vi "FollowPath.vi"(1 "Parameter String":string, 2 "Reinit":bool) -> (0 "Increment":bool)   [LabVIEW 2018]
uses:
  sensors.vi
  refnums.vi
  <vilib>/Rock Robotics/WPI/Utilities/WPI_GetSetVariantRefNum.vi
  dsinstructions.vi
panel:
  out "Robot Position":cluster{dbl[], dbl[]}[](graph)
  in  "Plot":bool
  in  "N-Int":i32=50
  in  "N-Diff":i32=50
  in  "Kd":dbl=1e-06
  in  "Ki":dbl=5e-06
  in  "Kp":dbl=3e-05
  out "Orientation PID Tracking":cluster{"Goal Wheel Position":dbl, dbl}(graph)={"Goal Wheel Position"=0.0, -90.17571233858979}
  out "Orientation Contribution Tracking":cluster{dbl, dbl, dbl}(graph)
  in  "Manual Control":bool=TRUE
  in  "Look-Ahead Time (s)":dbl=0.25
  in  "Search Window (s)":dbl=2.0
  # "Orientation Control"
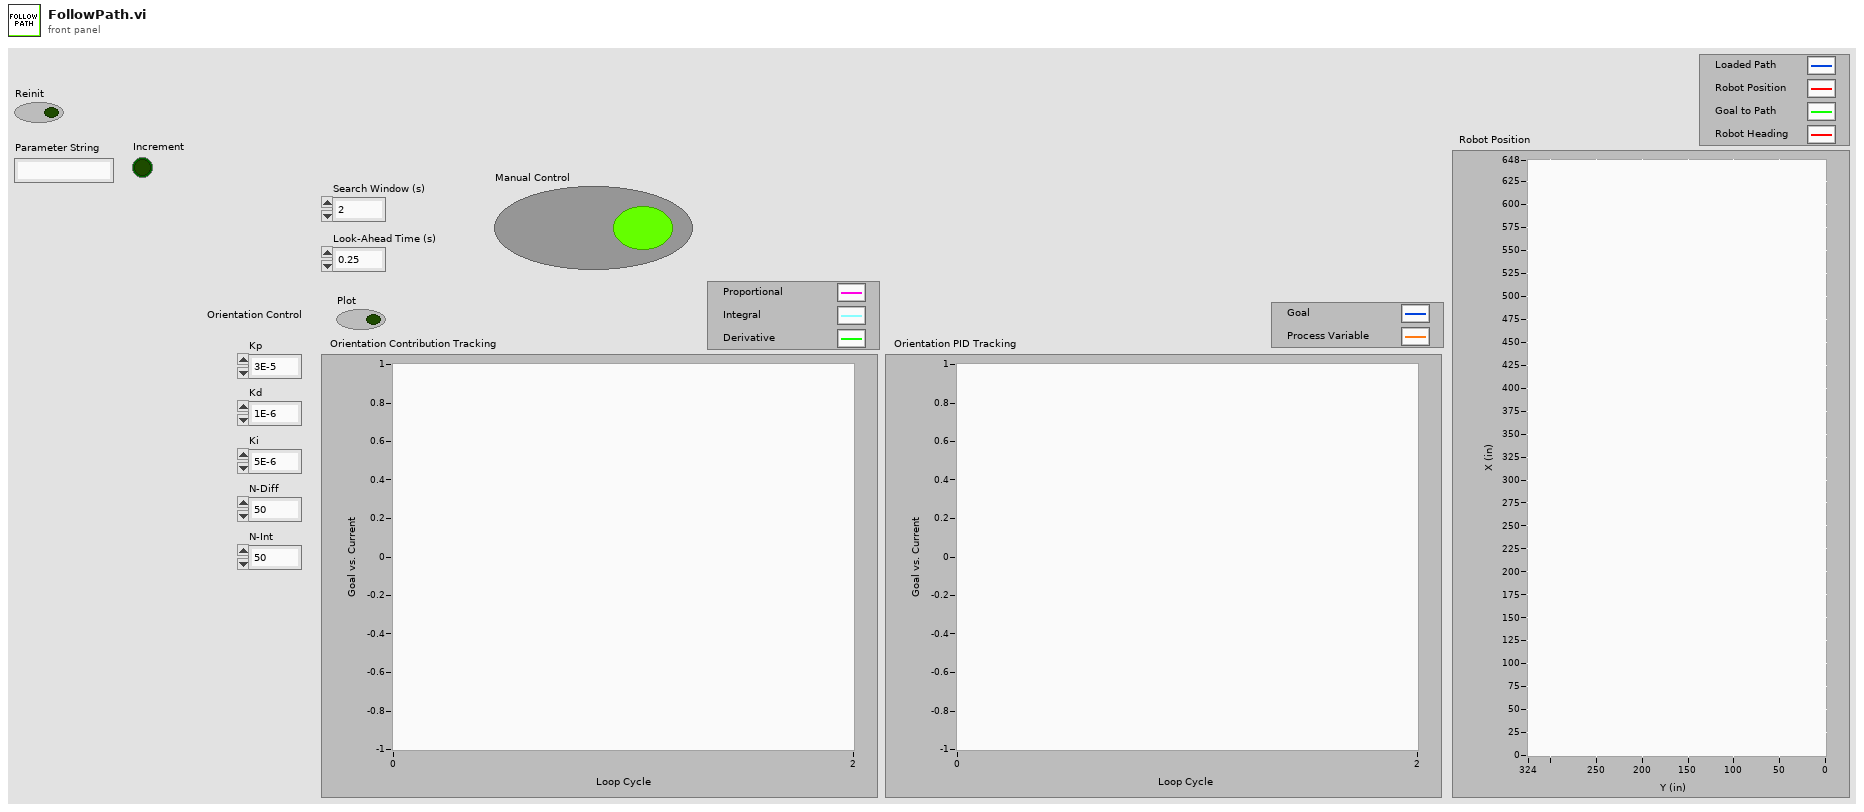
[diagram p1: front panel]
types:
  T1 = typedef "WPI_JoystickDevRef.ctl" = cluster{"Device":T2}
  T2 = typedef "WPI_JoystickDeviceEnum.ctl" = enum16{"USB 0", "USB 1", "USB 2", "USB 3", "USB 4", "USB 5"}
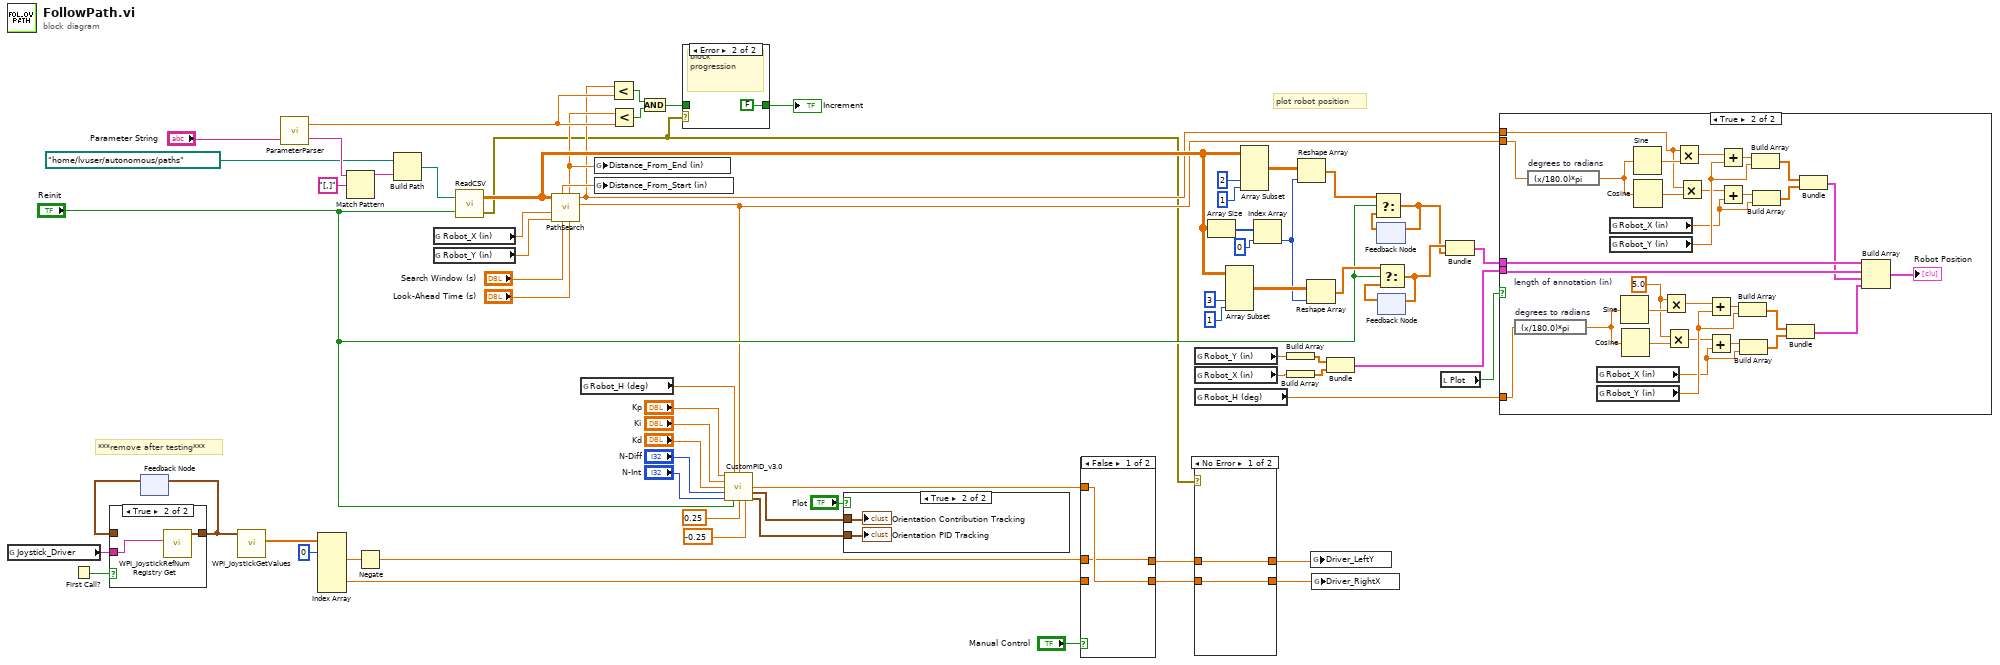
[diagram p0: block diagram]
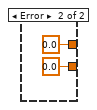
[diagram p3: hidden frame]
diagram:
  # "***remove after testing***"
  # "plot robot position"
  n1 = global read "refnums.vi" "Joystick_Driver"() -> (w57:string)
  n2 = First Call?() -> (First Call?: T/F=w60:bool)
  n3 = feedback #1() -> (w59:T1)  [unwired: 1 in]
  n4 = case shown="True" w60 {
    tunnel: [w72 w74] -> w58
    tunnel: w59 -> [w72 _]
    tunnel: w57 -> [_ w73]
    frame False {
    }
    frame True {
      n5 = call <vilib>:"WPI_JoystickRefNum Registry Get.vi"("refnum name"=w73) -> ("JoystickDevRef"=w74:T1)  [unwired: 9 in, 1 out]
    }
  }
  n6 = feedback-in #1(w58) -> ()
  n7 = call <vilib>:"WPI_JoystickGetValues.vi"("JoystickDevRef"=w58) -> ("Axes"=w56:dbl[])  [unwired: 6 in, 4 out]
  n8 = call "ParameterParser.vi"("Parameter String"="Parameter String") -> ("Remaining Parameter String"=w69:string, "Parameter"=w11:dbl)  [unwired: 1 in]
  n9 = Index Array(array=w56, index #1=0 ("index")) -> (element #2=w54:dbl, element #5=w52:dbl)  [unwired: 5 in, 4 out]
  n10 = Match Pattern(string=w69, regular expression="[,]") -> (before substring=w68:string)  [unwired: 1 in, 3 out]
  n11 = Negate(x=w54) -> (-x=w53:dbl)
  n12 = Build Path(base path=path "/home/lvuser/autonomous/paths" ("path"), name or relative path=w68) -> (appended path=w66:path)
  n13 = global read "sensors.vi" "Robot_X (in)"() -> (w64:dbl)
  n14 = global read "sensors.vi" "Robot_Y (in)"() -> (w63:dbl)
  n15 = call "ReadCSV.vi"("Reinit"="Reinit", "File Path (.csv)"=w66) -> ("File Open Eror"=w4:errorcluster, "Data (index by row)"=w26:dbl[][])
  n16 = call "PathSearch.vi"("Look-Ahead Time (s)"="Look-Ahead Time (s)", "Search Window (s)"="Search Window (s)", "Robot Y (in)"=w63, "Robot X (in)"=w64, "Path"=w26) -> ("Angle To Goal (deg)"=w12:dbl, "Distance to Goal (in)"=w9:dbl, "Distance from End (in)"=w10:dbl, "Distance from Start (in)"=w65:dbl)  [unwired: 1 in, 2 out]
  n17 = global read "sensors.vi" "Robot_H (deg)"() -> (w50:dbl)
  n18 = global write "sensors.vi" "Distance_From_End (in)"(w10) -> ()
  n19 = global write "sensors.vi" "Distance_From_Start (in)"(w65) -> ()
  n20 = Less?(x=w9, y=w11) -> (x < y?=w28:bool)
  n21 = Less?(x=w10, y=w11) -> (x < y?=w27:bool)
  n22 = And(x=w28, y=w27) -> (x .and. y?=w3:bool)
  n23 = case shown="Error" w4 {
    tunnel: [w75 FALSE] -> w2
    tunnel: w3 -> [w75 _]
    frame No Error {
    }
    frame Error {
      # "block progression"
    }
  }
  "Increment" <- w2
  n24 = call "CustomPID_v3.0.vi"("Kp"="Kp", "Process Variable"=w50, "Goal"=w12, "Ki"="Ki", "Kd"="Kd", "N-Diff"="N-Diff", "N-Int"="N-Int", "Reinit"="Reinit", "Max Ouput"=0.25, "Min Output"=-0.25) -> ("Command"=w49:dbl, "Contribution Tracking"=w48:cluster{dbl, dbl, dbl}, "PID Tracking"=w47:cluster{"Goal Wheel Position":dbl, dbl})  [unwired: 2 in, 1 out]
  n25 = case shown="True" "Plot" {
    tunnel: w48 -> [_ w78]
    tunnel: w47 -> [_ w77]
    frame False {
    }
    frame True {
      "Orientation Contribution Tracking" <- w78
      "Orientation PID Tracking" <- w77
    }
  }
  n26 = case shown="False" "Manual Control" {
    tunnel: [w79 w82] -> w8
    tunnel: w53 -> [w79 w82]
    tunnel: w52 -> [_ w81]
    tunnel: [w80 w81] -> w6
    tunnel: w49 -> [w80 _]
    frame False {
    }
    frame True {
    }
  }
  n27 = global read "sensors.vi" "Robot_Y (in)"() -> (w25:dbl)
  n28 = global read "sensors.vi" "Robot_X (in)"() -> (w24:dbl)
  n29 = global read "sensors.vi" "Robot_H (deg)"() -> (w1:dbl)
  n30 = case shown="No Error" w4 {
    tunnel: [w84 0.0] -> w7
    tunnel: w8 -> [w84 _]
    tunnel: [w83 0.0 ("upper limit")] -> w5
    tunnel: w6 -> [w83 _]
    frame No Error {
    }
    frame Error {
    }
  }
  n31 = Array Size(array=w26) -> (size(s)=w31:i32[])
  n32 = Array Subset(array=w26, index (col)=3 ("index"), length (col)=1 ("length")) -> (w32:dbl[][])  [unwired: 2 in]
  n33 = Array Subset(array=w26, index (col)=2 ("index"), length (col)=1 ("length")) -> (w34:dbl[][])  [unwired: 2 in]
  n34 = Index Array(array=w31, index=0) -> (element=w29:i32)
  n35 = Build Array(w25) -> (w22:dbl[])
  n36 = Build Array(w24) -> (w23:dbl[])
  n37 = Reshape Array(w34, w29) -> (w14:dbl[])
  n38 = Reshape Array(w32, w29) -> (w33:dbl[])
  n39 = global write "dsinstructions.vi" "Driver_LeftY"(w7) -> ()
  n40 = global write "dsinstructions.vi" "Driver_RightX"(w5) -> ()
  n41 = Bundle(w22, w23) -> (w17:cluster{dbl[], dbl[]})  [unwired: 1 in]
  n42 = feedback #2() -> (w19:dbl[])  [unwired: 1 in]
  n43 = Select(t=w14, s="Reinit", f=w19) -> (s? t:f=w20:dbl[])
  n44 = feedback-in #2(w20) -> ()
  n45 = feedback #3() -> (w18:dbl[])  [unwired: 1 in]
  n46 = Select(t=w33, s="Reinit", f=w18) -> (s? t:f=w21:dbl[])
  n47 = feedback-in #3(w21) -> ()
  n48 = local read "Plot"() -> (w13:bool)
  n49 = Bundle(w21, w20) -> (w16:cluster{dbl[], dbl[]})  [unwired: 1 in]
  n50 = case shown="True" w13 {
    tunnel: w17 -> [_ w116]
    tunnel: w16 -> [_ w115]
    tunnel: w9 -> [_ w103]
    tunnel: w12 -> [_ w102]
    tunnel: w1 -> [_ w89]
    frame False {
    }
    frame True {
      w88 = 5.0  # length of annotation (in)
      n51 = expression code="(x/180.0)*pi" "degrees to radians"(w89) -> (w90:dbl)
      n52 = expression code="(x/180.0)*pi" "degrees to radians"(w102) -> (w104:dbl)
      n53 = global read "sensors.vi" "Robot_X (in)"() -> (w99:dbl)
      n54 = global read "sensors.vi" "Robot_Y (in)"() -> (w100:dbl)
      n55 = global read "sensors.vi" "Robot_X (in)"() -> (w113:dbl)
      n56 = global read "sensors.vi" "Robot_Y (in)"() -> (w114:dbl)
      n57 = Sine(x=w90) -> (sin(x)=w91:dbl)
      n58 = Cosine(x=w90) -> (cos(x)=w92:dbl)
      n59 = Sine(x=w104) -> (sin(x)=w105:dbl)
      n60 = Cosine(x=w104) -> (cos(x)=w106:dbl)
      n61 = Multiply(x=w88, y=w91) -> (x*y=w93:dbl)
      n62 = Multiply(x=w88, y=w92) -> (x*y=w94:dbl)
      n63 = Multiply(x=w103, y=w105) -> (x*y=w107:dbl)
      n64 = Multiply(x=w103, y=w106) -> (x*y=w108:dbl)
      n65 = Add(x=w93, y=w100) -> (x+y=w95:dbl)
      n66 = Add(x=w94, y=w99) -> (x+y=w96:dbl)
      n67 = Add(x=w107, y=w114) -> (x+y=w109:dbl)
      n68 = Add(x=w108, y=w113) -> (x+y=w110:dbl)
      n69 = Build Array(w95, w100) -> (w97:dbl[])
      n70 = Build Array(w96, w99) -> (w98:dbl[])
      n71 = Build Array(w109, w114) -> (w111:dbl[])
      n72 = Build Array(w110, w113) -> (w112:dbl[])
      n73 = Bundle(w97, w98) -> (w87:cluster{dbl[], dbl[]})  [unwired: 1 in]
      n74 = Bundle(w111, w112) -> (w101:cluster{dbl[], dbl[]})  [unwired: 1 in]
      n75 = Build Array(w115, w116, w101, w87) -> (→"Robot Position":cluster{dbl[], dbl[]}[])
    }
  }
